vi "Fit parameters chooser.vi"(0 "Stop signaller":refnum<class "Signaller.lvclass">, 5 "Fit parameters refnum":refnum<vi>, 7 "C refnum":refnum<vi>, 9 "Physical constants refnum":refnum<vi>, 11 "Simulation parameters semaphore":T1) -> ()   [LabVIEW 2019]
uses:
  Fit Parameters.ctl
  Physical Constants.ctl
  Motor controller/Signaller/Signaller.lvclass
  <vilib>/gmath/statdist.llb/Continuous PDF.vi
  <vilib>/gmath/statdist.llb/Normal PDF.vi
  <vilib>/gmath/NI_Gmath.lvlib
  <vilib>/Utility/config.llb/NI_LVConfig.lvlib
panel:
  out "Optimal steady state (negative)":dbl format="%.3g"
  out "Optimal steady state (positive)":dbl format="%.3g"
  out "Optimal frequency (negative) (GHz)":dbl format="%.3g"
  out "Optimal frequency (positive) (GHz)":dbl format="%.3g"
  in  "Overwrite selected preset":bool
  in  "Save as new preset":bool
  in  "Load from preset":bool
  in  "Choose preset":u16(ring) items=["ND-3", "new_pro", "NH3", "sharp", "Test", "test2"]
  in  "Refresh graphs":bool
  in  "Update simulation parameters":bool
  in  "Physical constants":T2={"T1e (s)"=0.03, "T1n (s)"=1500.0}
  in  "C":dbl=0.000136073
  in  "Fit parameters":T3={"A"=0.572086, "S"=0.0835606, "M1"=140.286, "M2"=140.486}
  out "Steady state distribution":cluster{dbl[], dbl[]}(graph)
  out "Alpha/beta distributions":cluster{dbl[], dbl[]}[](graph)
  # "Explanation of fit parameters:\nThe parameters A, S, M1, and M2 control the distribution of alpha and beta as shown above. The steady state distribution will be computed from these.\nA: the height of the Gaussian distributions for alpha and beta\nS: the standard deviation of the Gaussian distributions for alpha and beta\nM1: the mean of the Gaussian distribution for beta\nM2: the mean of the Gaussian distribution for alpha"
  # "Internal controls"
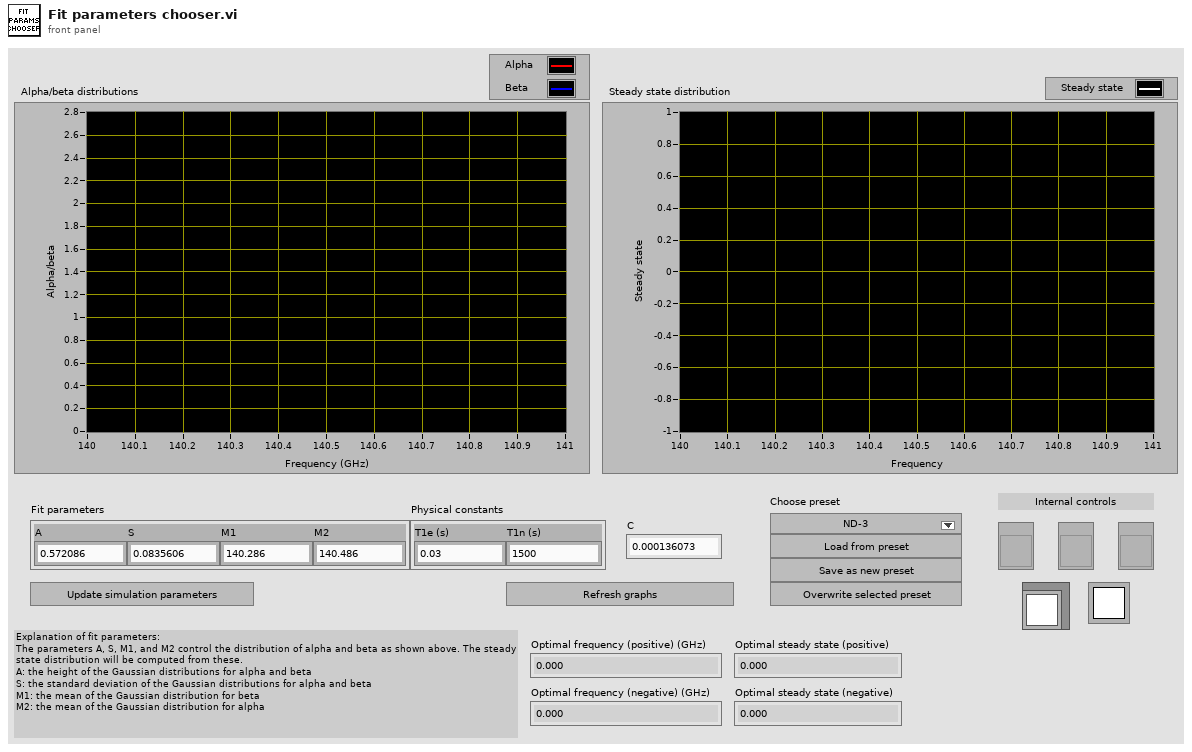
[diagram p1: front panel]
types:
  T1 = typedef "Semaphore RefNum" = refnum<k1>
  T2 = typedef "Physical Constants.ctl" = cluster{"T1e (s)":dbl, "T1n (s)":dbl}
  T3 = typedef "Fit Parameters.ctl" = cluster{"A":dbl, "S":dbl, "M1":dbl, "M2":dbl}
  T4 = typedef "LVRangeTypeDef.ctl" = cluster{"Minimum":dbl, "Maximum":dbl, "Increment":dbl, "Minor Increment":dbl, "Start":dbl}
  T5 = enum8{"Enabled", "Disabled", "Disabled and Grayed Out"}
  T6 = typedef "fit_parameters.ctl" = cluster{"A":dbl, "S":dbl, "M1":dbl, "M2":dbl}
  T7 = typedef "physical_constants.ctl" = cluster{"T1e (s)":dbl, "T1n (s)":dbl}
  T8 = typedef "NI_LVConfig.lvlib/Config Data RefNum.ctl" = refnum<k1>
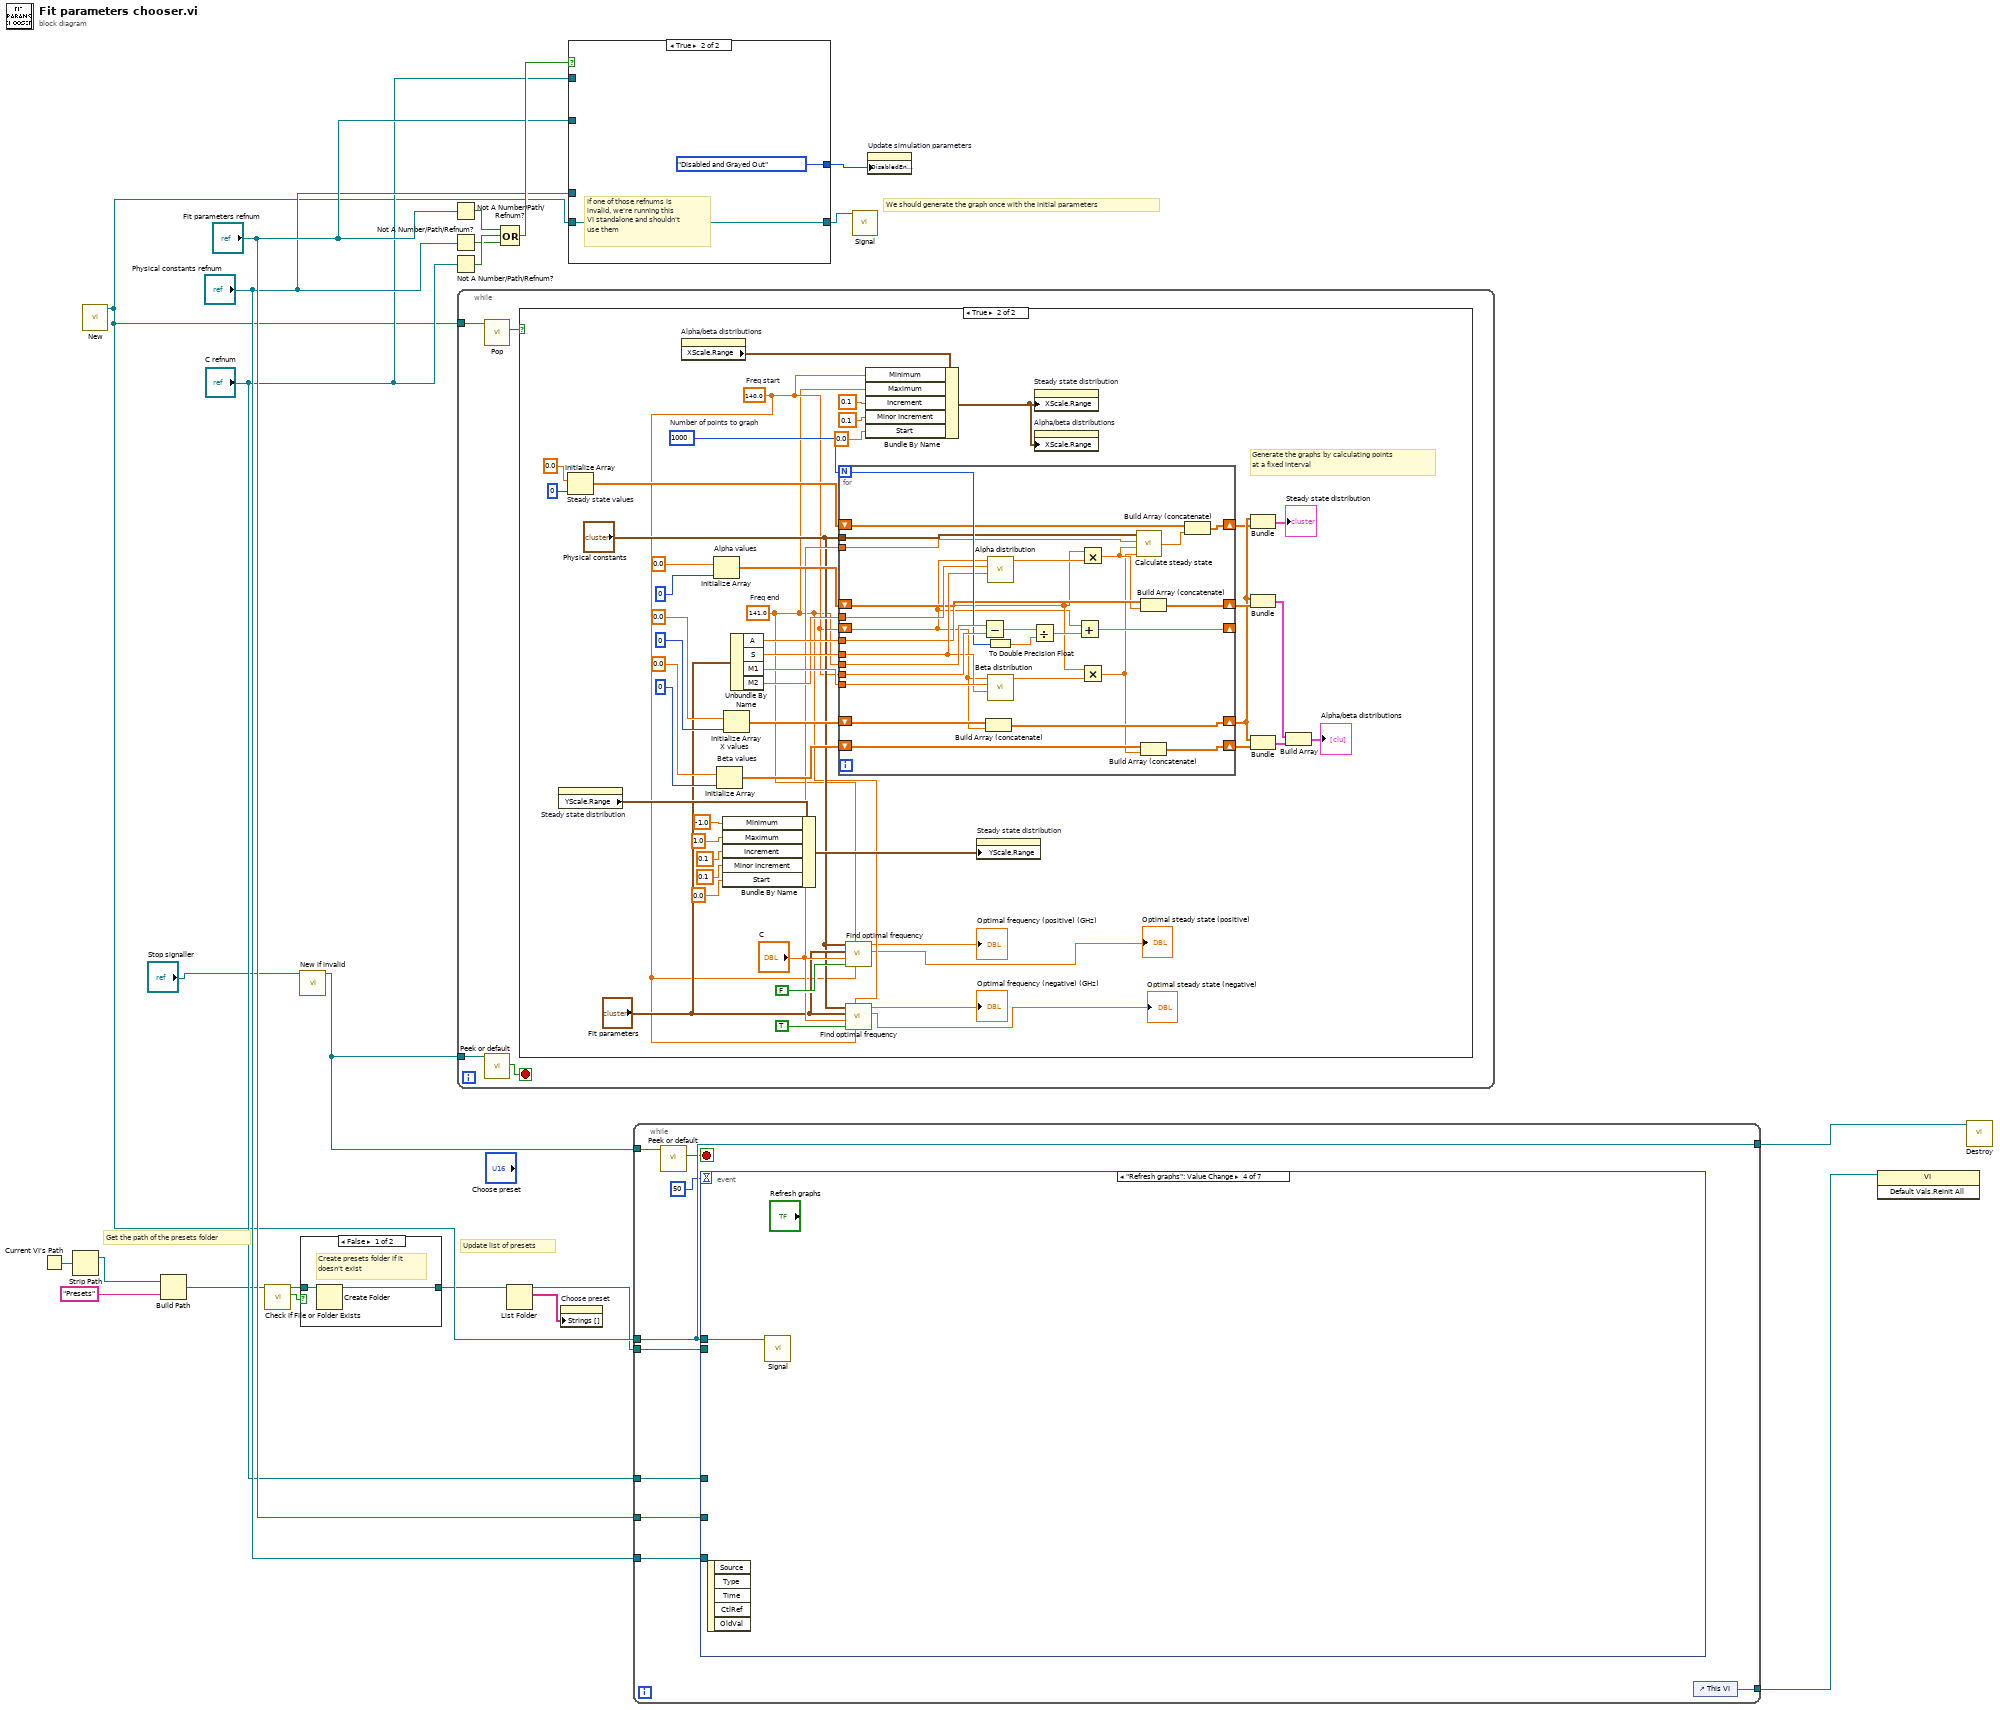
[diagram p0: block diagram]
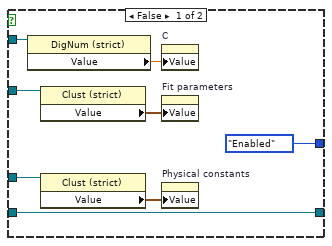
[diagram p3: hidden frame]
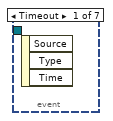
[diagram p4: hidden frame]
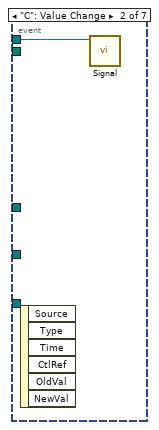
[diagram p5: hidden frame]
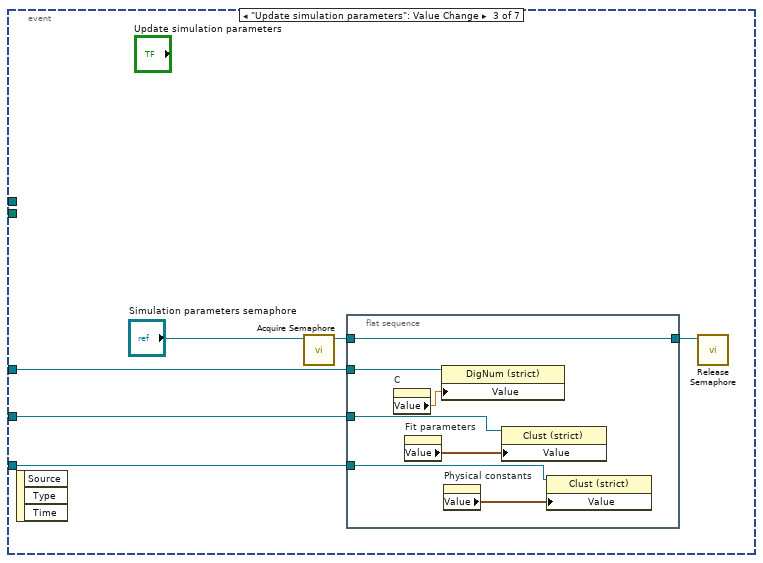
[diagram p6: hidden frame]
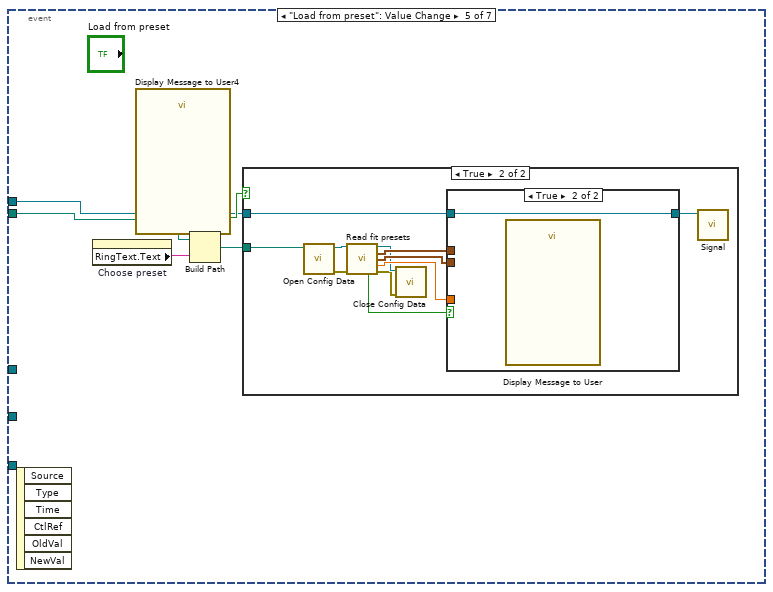
[diagram p7: hidden frame]
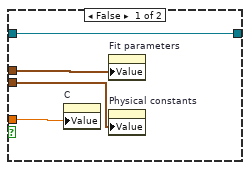
[diagram p9: hidden frame]
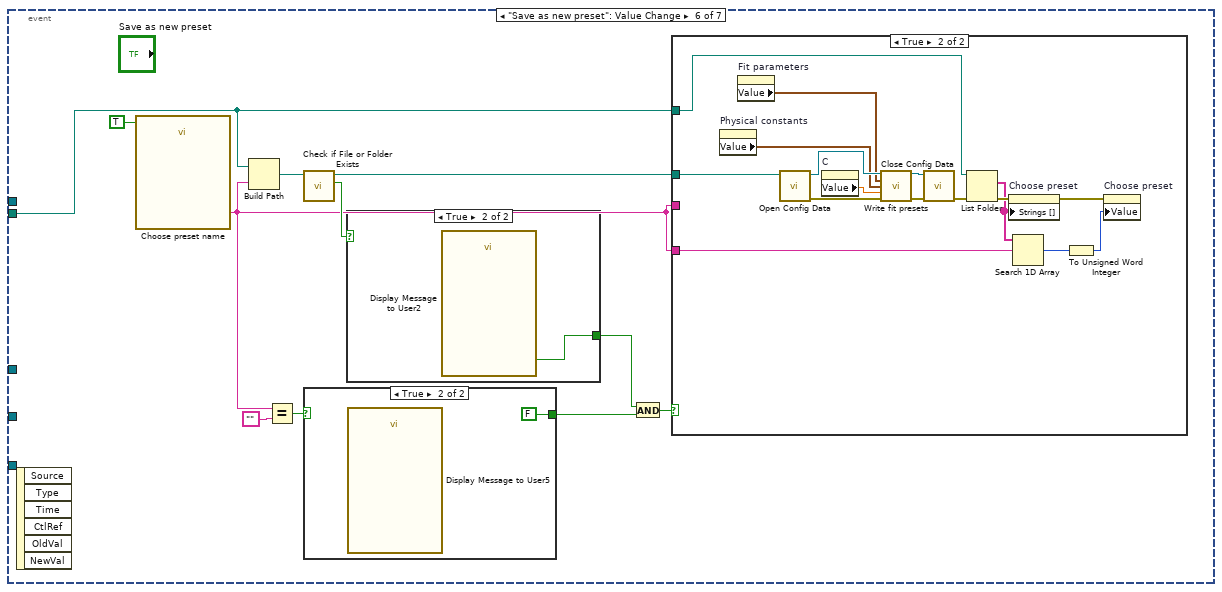
[diagram p10: hidden frame]
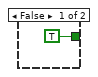
[diagram p11: hidden frame]
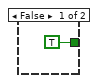
[diagram p13: hidden frame]
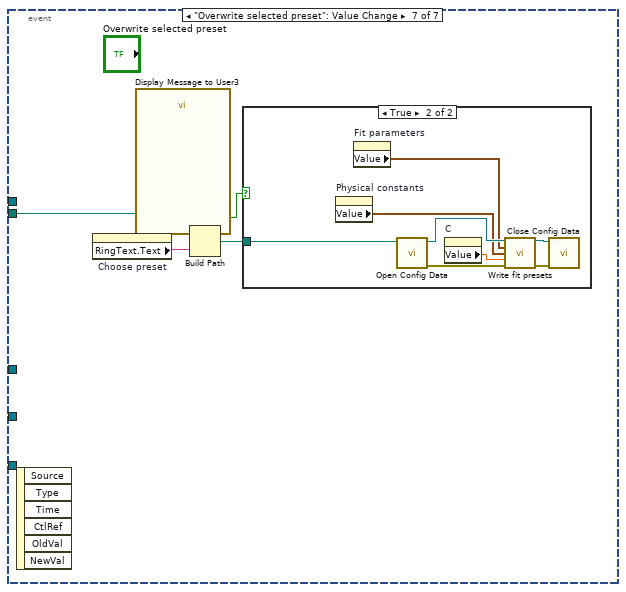
[diagram p14: hidden frame]
diagram:
  # "Update list of presets"
  # "Get the path of the presets folder"
  # "We should generate the graph once with the initial parameters"
  n1 = Current VI's Path() -> (path=w8:path)
  n2 = Strip Path(path=w8) -> (stripped path=w9:path)  [unwired: 1 out]
  n3 = call "New.vi"() -> ("Signaller out"=w12:refnum<class "Signaller.lvclass">)  [unwired: 11 in]
  n4 = Build Path(base path=w9, name or relative path="Presets") -> (appended path=w7:path)
  n5 = call <vilib>:"Check if File or Folder Exists.vi"("path"=w7) -> ("file or folder exists?"=w6:bool, "dup path"=w5:path)  [unwired: 8 in, 1 out]
  n6 = call "New if invalid.vi"("Signaller in"="Stop signaller") -> ("Signaller out"=w11:refnum<class "Signaller.lvclass">)  [unwired: 9 in, 1 out]
  n7 = case shown="False" w6 {
    tunnel: w5 -> [w25 w26]
    tunnel: [w24 w26] -> w4
    frame False {
      # "Create presets folder if it\ndoesn't exist"
      n8 = Create Folder(path (use dialog)=w25) -> (created path=w24:path)  [unwired: 2 in, 2 out]
    }
    frame True {
    }
  }
  n9 = Not A Number/Path/Refnum?(number/path/refnum="Fit parameters refnum") -> (NaN/Path/Refnum?=w21:bool)
  n10 = Not A Number/Path/Refnum?(number/path/refnum="Physical constants refnum") -> (NaN/Path/Refnum?=w19:bool)
  n11 = Not A Number/Path/Refnum?(number/path/refnum="C refnum") -> (NaN/Path/Refnum?=w20:bool)
  n12 = while {
    tunnel: w12 -> [w29]
    tunnel: w11 -> [w28]
    stop <- w27 stop-if-true
    n13 = call "Pop.vi"("Signaller in"=w29) -> ("Has signal"=w30:bool)  [unwired: 8 in, 2 out]
    n14 = call "Peek or default.vi"("Signaller in"=w28) -> ("Has signal?"=w27:bool)  [unwired: 8 in, 2 out]
    n15 = case shown="True" w30 {
      frame False {
      }
      frame True {
        w35 = 141.0  # Freq end
        w36 = 140.0  # Freq start
        w78 = 1000  # Number of points to graph
        # "Generate the graphs by calculating points\nat a fixed interval"
        n16 = property on="Steady state distribution" class="XYGraph (strict)"() -> ("YScale.Range"=w48:T4)  [unwired: 2 in, 2 out]
        n17 = Initialize Array "Steady state values"(0.0 ("element"), 0 ("dimension size")) -> (w52:dbl[])
        n18 = property on="Alpha/beta distributions" class="XYGraph (strict)"() -> ("XScale.Range"=w74:T4)  [unwired: 2 in, 2 out]
        n19 = Initialize Array "Alpha values"(0.0 ("element"), 0 ("dimension size")) -> (w61:dbl[])
        n20 = Initialize Array "Beta values"(0.0 ("element"), 0 ("dimension size")) -> (w62:dbl[])
        n21 = Bundle By Name(cluster=w48, "Minimum"=-1.0, "Maximum"=1.0, "Increment"=0.1, "Minor Increment"=0.1, "Start"=0.0) -> (w47:T4)
        n22 = Initialize Array "X values"(0.0 ("element"), 0 ("dimension size")) -> (w67:dbl[])
        n23 = Unbundle By Name("Fit parameters") -> ("A"=w77:dbl, "S"=w75:dbl, "M1"=w76:dbl, "M2"=w70:dbl)
        n24 = for {
          N: w78 -> [w99]
          shift-right: [w97] -> _
          shift-left: w36 -> [w86]
          tunnel: w77 -> [w90]
          tunnel: w76 -> [w104]
          tunnel: w75 -> [w95]
          tunnel: w35 -> [w103]
          tunnel: w36 -> [w102]
          tunnel: w70 -> [w96]
          shift-right: [w87] -> w51
          shift-left: w67 -> [w94]
          shift-right: [w89] -> w59
          shift-left: w62 -> [w92]
          shift-right: [w88] -> w60
          shift-left: w61 -> [w93]
          shift-right: [w83] -> w50
          shift-left: w52 -> [w85]
          tunnel: "Physical constants" -> [w82]
          tunnel: "C" -> [w81]
          n25 = Subtract(x=w103, y=w102) -> (x-y=w101:dbl)
          n26 = Build Array (concatenate)(w94, w86) -> (w87:dbl[])
          n27 = call-poly "Alpha distribution"("std"=w95, "mean"=w96, "x"=w86) -> ("pdf(x)"=w91:dbl)  [unwired: 7 in, 1 out]
          n28 = To Double Precision Float(number=w99) -> (double precision float=w100:dbl)
          n29 = call-poly "Beta distribution"("std"=w95, "mean"=w104, "x"=w86) -> ("pdf(x)"=w105:dbl)  [unwired: 7 in, 1 out]
          n30 = Divide(x=w101, y=w100) -> (x/y=w98:dbl)
          n31 = Add(x=w86, y=w98) -> (x+y=w97:dbl)
          n32 = Multiply(x=w90, y=w91) -> (x*y=w80:dbl)
          n33 = Multiply(x=w90, y=w105) -> (x*y=w79:dbl)
          n34 = call "Calculate steady state.vi"("Beta"=w79, "Alpha"=w80, "C"=w81, "Physical constants"=w82) -> ("Steady state"=w84:dbl)
          n35 = Build Array (concatenate)(w93, w80) -> (w88:dbl[])
          n36 = Build Array (concatenate)(w92, w79) -> (w89:dbl[])
          n37 = Build Array (concatenate)(w85, w84) -> (w83:dbl[])
        }
        n38 = call "Find optimal frequency.vi"("Bottom end of range (GHz) (140.0)"=w36, "Top end of range (GHz) (141.0)"=w35, "Find optimal for negative polarization?"=FALSE, "C"="C", "Fit parameters"="Fit parameters", "Physical constants"="Physical constants") -> ("Steady state at optimal frequency"=→"Optimal steady state (positive)":dbl, "Optimal frequency (GHz)"=→"Optimal frequency (positive) (GHz)":dbl)  [unwired: 4 in]
        n39 = call "Find optimal frequency.vi"("Bottom end of range (GHz) (140.0)"=w36, "Top end of range (GHz) (141.0)"=w35, "Find optimal for negative polarization?"=TRUE, "C"="C", "Fit parameters"="Fit parameters", "Physical constants"="Physical constants") -> ("Steady state at optimal frequency"=→"Optimal steady state (negative)":dbl, "Optimal frequency (GHz)"=→"Optimal frequency (negative) (GHz)":dbl)  [unwired: 4 in]
        n40 = Bundle By Name(cluster=w74, "Minimum"=w36, "Maximum"=w35, "Increment"=0.1, "Minor Increment"=0.1, "Start"=0.0) -> (w55:T4)
        n41 = property on="Steady state distribution" class="XYGraph (strict)"("YScale.Range"=w47) -> ()  [unwired: 2 in, 2 out]
        n42 = property on="Steady state distribution" class="XYGraph (strict)"("XScale.Range"=w55) -> ()  [unwired: 2 in, 2 out]
        n43 = property on="Alpha/beta distributions" class="XYGraph (strict)"("XScale.Range"=w55) -> ()  [unwired: 2 in, 2 out]
        n44 = Bundle(w51, w50) -> (→"Steady state distribution":cluster{dbl[], dbl[]})  [unwired: 1 in]
        n45 = Bundle(w51, w60) -> (w58:cluster{dbl[], dbl[]})  [unwired: 1 in]
        n46 = Bundle(w51, w59) -> (w57:cluster{dbl[], dbl[]})  [unwired: 1 in]
        n47 = Build Array(w58, w57) -> (→"Alpha/beta distributions":cluster{dbl[], dbl[]}[])
      }
    }
  }
  n48 = Compound Arithmetic op=OR(w21, w20, w19) -> (w22:bool)
  n49 = List Folder(path=w4) -> (path out=w2:path, filenames=w3:string[])  [unwired: 3 in, 2 out]
  n50 = property on="Choose preset" class="Ring (strict)"("Strings []"=w3) -> ()  [unwired: 2 in, 2 out]
  n51 = case shown="True" w22 {
    tunnel: [T5."Enabled" ("Disabled") T5."Disabled and Grayed Out" ("Disabled")] -> w18
    tunnel: "Fit parameters refnum" -> [w112 _]
    tunnel: "C refnum" -> [w110 _]
    tunnel: "Physical constants refnum" -> [w109 _]
    tunnel: w12 -> [w106 w114]
    tunnel: [w106 w114] -> w17
    frame False {
      n52 = property class="DigNum (strict)"(reference=w110) -> ("Value"=w108:dbl)  [unwired: 1 in, 2 out]
      n53 = property class="Clust (strict)"(reference=w112) -> ("Value"=w111:T6)  [unwired: 1 in, 2 out]
      n54 = property class="Clust (strict)"(reference=w109) -> ("Value"=w107:T7)  [unwired: 1 in, 2 out]
      n55 = property on="C" class="DigNum (strict)"("Value"=w108) -> ()  [unwired: 2 in, 2 out]
      n56 = property on="Fit parameters" class="Clust (strict)"("Value"=w111) -> ()  [unwired: 2 in, 2 out]
      n57 = property on="Physical constants" class="Clust (strict)"("Value"=w107) -> ()  [unwired: 2 in, 2 out]
    }
    frame True {
      # "If one of those refnums is\ninvalid, we're running this\nVI standalone and shouldn't\nuse them"
    }
  }
  n58 = while {
    tunnel: w12 -> [w124]
    tunnel: [w124] -> w23
    tunnel: "Fit parameters refnum" -> [w123]
    tunnel: "Physical constants refnum" -> [w122]
    tunnel: "C refnum" -> [w121]
    tunnel: w11 -> [w119]
    tunnel: w2 -> [w117]
    tunnel: [w116] -> w1
    stop <- w120 stop-if-true
    n59 = call "Peek or default.vi"("Signaller in"=w119) -> ("Has signal?"=w120:bool)  [unwired: 8 in, 2 out]
    n60 = event shown="[3] \"Refresh graphs\": Value Change" {
      selector: _ -> [_ _ _ _ _ _ _]
      dyn-events: _ -> [_ _ _ _ _ _ _]
      timeout: 50 -> [_ _ _ _ _ _ _]
      tunnel: w124 -> [_ w125 _ w139 w140 _ _]
      tunnel: w123 -> [_ _ w131 _ _ _ _]
      tunnel: w122 -> [_ _ w130 _ _ _ _]
      tunnel: w121 -> [_ _ w129 _ _ _ _]
      tunnel: w117 -> [_ _ _ _ w144 w168 w195]
      event Timeout {
        n61 = event-data() -> ()  [unwired: 1 in, 3 out]
      }
      event "C": Value Change {
        n62 = event-data() -> ()  [unwired: 1 in, 6 out]
        n63 = call "Signal.vi"("Signaller in"=w125) -> ()  [unwired: 9 in, 2 out]
      }
      event "Update simulation parameters": Value Change {
        n64 = event-data() -> ()  [unwired: 1 in, 3 out]
        n65 = call <vilib>:"Acquire Semaphore.vi"("semaphore"="Simulation parameters semaphore") -> ("semaphore out"=w127:T1)  [unwired: 4 in, 2 out]
        n66 = flat-sequence {
          tunnel: w131 -> [w138]
          tunnel: w130 -> [w137]
          tunnel: w129 -> [w136]
          tunnel: w127 -> [w132]
          tunnel: [w132] -> w126
          frame #0 {
            n67 = property on="C" class="DigNum (strict)"() -> ("Value"=w133:dbl)  [unwired: 2 in, 2 out]
            n68 = property on="Fit parameters" class="Clust (strict)"() -> ("Value"=w135:T3)  [unwired: 2 in, 2 out]
            n69 = property class="DigNum (strict)"(reference=w136, "Value"=w133) -> ()  [unwired: 1 in, 2 out]
            n70 = property on="Physical constants" class="Clust (strict)"() -> ("Value"=w134:T2)  [unwired: 2 in, 2 out]
            n71 = property class="Clust (strict)"(reference=w138, "Value"=w135) -> ()  [unwired: 1 in, 2 out]
            n72 = property class="Clust (strict)"(reference=w137, "Value"=w134) -> ()  [unwired: 1 in, 2 out]
          }
        }
        n73 = call <vilib>:"Release Semaphore.vi"("semaphore"=w126) -> ()  [unwired: 5 in, 2 out]
      }
      event "Refresh graphs": Value Change {
        n74 = event-data() -> ()  [unwired: 1 in, 5 out]
        n75 = call "Signal.vi"("Signaller in"=w139) -> ()  [unwired: 9 in, 2 out]
      }
      event "Load from preset": Value Change {
        n76 = event-data() -> ()  [unwired: 1 in, 6 out]
        n77 = property on="Choose preset" class="Ring (strict)"() -> ("RingText.Text"=w143:string)  [unwired: 2 in, 2 out]
        n78 = call "Display Message to User4"() -> ("Yes"=w141:bool)  [unwired: 10 in, 1 out]
        n79 = Build Path(base path=w144, name or relative path=w143) -> (appended path=w142:path)
        n80 = case shown="True" w141 {
          tunnel: w142 -> [_ w155]
          tunnel: w140 -> [_ w146]
          frame False {
          }
          frame True {
            n81 = call <vilib>:"Open Config Data.vi"("configuration file path"=w155) -> ("error out"=w148:errorcluster, "refnum"=w154:T8)  [unwired: 8 in, 1 out]
            n82 = call "Read fit presets.vi"("Config file in"=w154, "error in (no error)"=w148) -> ("Config file out"=w149:T8, "Fit parameters"=w153:T3, "Physical constants"=w152:T2, "C"=w151:dbl, "Key not found?"=w150:bool, "error out"=w147:errorcluster)  [unwired: 8 in]
            n83 = call <vilib>:"Close Config Data.vi"("error in (no error)"=w147, "refnum"=w149) -> ()  [unwired: 8 in, 2 out]
            n84 = case shown="True" w150 {
              tunnel: w153 -> [w159 _]
              tunnel: w152 -> [w158 _]
              tunnel: w151 -> [w157 _]
              tunnel: w146 -> [w156 w160]
              tunnel: [w156 w160] -> w145
              frame False {
                n85 = property on="C" class="DigNum (strict)"("Value"=w157) -> ()  [unwired: 2 in, 2 out]
                n86 = property on="Fit parameters" class="Clust (strict)"("Value"=w159) -> ()  [unwired: 2 in, 2 out]
                n87 = property on="Physical constants" class="Clust (strict)"("Value"=w158) -> ()  [unwired: 2 in, 2 out]
              }
              frame True {
                n88 = call "Display Message to User"() -> ()  [unwired: 10 in, 2 out]
              }
            }
            n89 = call "Signal.vi"("Signaller in"=w145) -> ()  [unwired: 9 in, 2 out]
          }
        }
      }
      event "Save as new preset": Value Change {
        n90 = event-data() -> ()  [unwired: 1 in, 6 out]
        n91 = call "Choose preset name"("Enable"=TRUE) -> ("Preset name"=w165:string)  [unwired: 16 in, 2 out]
        n92 = Build Path(base path=w168, name or relative path=w165) -> (appended path=w171:path)
        n93 = Equal?(x=w165, y="") -> (x = y?=w164:bool)
        n94 = call <vilib>:"Check if File or Folder Exists.vi"("path"=w171) -> ("file or folder exists?"=w170:bool, "dup path"=w169:path)  [unwired: 8 in, 1 out]
        n95 = case shown="True" w164 {
          tunnel: [TRUE FALSE] -> w161
          frame False {
          }
          frame True {
            n96 = call "Display Message to User5"() -> ()  [unwired: 10 in, 2 out]
          }
        }
        n97 = case shown="True" w170 {
          tunnel: [TRUE ("Yes") w191] -> w162
          frame False {
          }
          frame True {
            n98 = call "Display Message to User2"() -> ("Yes"=w191:bool)  [unwired: 10 in, 1 out]
          }
        }
        n99 = And(x=w162, y=w161) -> (x .and. y?=w163:bool)
        n100 = case shown="True" w163 {
          tunnel: w169 -> [_ w189]
          tunnel: w165 -> [_ _]
          tunnel: w168 -> [_ w183]
          tunnel: w165 -> [_ w177]
          frame False {
          }
          frame True {
            n101 = property on="Physical constants" class="Clust (strict)"() -> ("Value"=w186:T2)  [unwired: 2 in, 2 out]
            n102 = property on="Fit parameters" class="Clust (strict)"() -> ("Value"=w187:T3)  [unwired: 2 in, 2 out]
            n103 = call <vilib>:"Open Config Data.vi"("configuration file path"=w189) -> ("error out"=w181:errorcluster, "refnum"=w188:T8)  [unwired: 8 in, 1 out]
            n104 = property on="C" class="DigNum (strict)"() -> ("Value"=w185:dbl)  [unwired: 2 in, 2 out]
            n105 = call "Write fit presets.vi"("Config file in"=w188, "Fit parameters"=w187, "Physical constants"=w186, "C"=w185, "error in (no error)"=w181) -> ("Config file out"=w184:T8, "error out"=w180:errorcluster)  [unwired: 9 in]
            n106 = call <vilib>:"Close Config Data.vi"("error in (no error)"=w180, "refnum"=w184) -> ("error out"=w182:errorcluster)  [unwired: 8 in, 1 out]
            n107 = List Folder(path=w183, error in=w182) -> (filenames=w178:string[], error out=w179:errorcluster)  [unwired: 2 in, 2 out]
            n108 = property on="Choose preset" class="Ring (strict)"(error in=w179, "Strings []"=w178) -> (error out=w174:errorcluster)  [unwired: 1 in, 1 out]
            n109 = Search 1D Array(1D array=w178, element=w177) -> (index of element=w176:i32)  [unwired: 1 in]
            n110 = To Unsigned Word Integer(number=w176) -> (unsigned 16bit integer=w175:u16)
            n111 = property on="Choose preset" class="Ring (strict)"(error in=w174, "Value"=w175) -> ()  [unwired: 1 in, 2 out]
          }
        }
      }
      event "Overwrite selected preset": Value Change {
        n112 = event-data() -> ()  [unwired: 1 in, 6 out]
        n113 = property on="Choose preset" class="Ring (strict)"() -> ("RingText.Text"=w194:string)  [unwired: 2 in, 2 out]
        n114 = call "Display Message to User3"() -> ("Yes"=w193:bool)  [unwired: 10 in, 1 out]
        n115 = Build Path(base path=w195, name or relative path=w194) -> (appended path=w192:path)
        n116 = case shown="True" w193 {
          tunnel: w192 -> [_ w203]
          frame False {
          }
          frame True {
            n117 = property on="Physical constants" class="Clust (strict)"() -> ("Value"=w200:T2)  [unwired: 2 in, 2 out]
            n118 = property on="Fit parameters" class="Clust (strict)"() -> ("Value"=w201:T3)  [unwired: 2 in, 2 out]
            n119 = call <vilib>:"Open Config Data.vi"("configuration file path"=w203) -> ("error out"=w197:errorcluster, "refnum"=w202:T8)  [unwired: 8 in, 1 out]
            n120 = property on="C" class="DigNum (strict)"() -> ("Value"=w199:dbl)  [unwired: 2 in, 2 out]
            n121 = call "Write fit presets.vi"("Config file in"=w202, "Fit parameters"=w201, "Physical constants"=w200, "C"=w199, "error in (no error)"=w197) -> ("Config file out"=w198:T8, "error out"=w196:errorcluster)  [unwired: 9 in]
            n122 = call <vilib>:"Close Config Data.vi"("error in (no error)"=w196, "refnum"=w198) -> ()  [unwired: 8 in, 2 out]
          }
        }
      }
    }
    n123 = control-ref of="This VI"() -> (w116:refnum<vi>)
  }
  n124 = call "Signal.vi"("Signaller in"=w17) -> ()  [unwired: 9 in, 2 out]
  n125 = property on="Update simulation parameters" class="Bool"("DisabledEnum"=w18) -> ()  [unwired: 2 in, 2 out]
  n126 = invoke class="VI" method="Default Vals.Reinit All"(reference=w1) -> ()  [unwired: 2 in, 3 out]
  n127 = call "Destroy.vi"("Signaller in"=w23) -> ()  [unwired: 10 in, 1 out]
